vi "Global_ACT Write_Data Out.vi"() -> ()   [LabVIEW 2017, in "Claw.lvlib"]
uses:
  Claw.lvlib
  <vilib>/Rock Robotics/WPI/Solenoid/WPI_SolenoidValue.ctl
  TypeDef/CLUSTER_Two Motor Output.ctl
  CLUSTER_Limit_Switch_Output.ctl
panel:
  in  "Claw_ACT_Limit_Switch":T1
  in  "Claw_ACT_Claw_Motors":T2
  in  "Claw_ACT_Piston_Output":T3
  # "The Names of the Data items in the Global Variable MUST describe who the Single Writer is\nNaming Convention of all Data Items is:   \nLib Name_Loop Name (SM or SEN or ACT)_Data Name\nExamples:\nDrive_ACT_X axis\nGameController_SEN_JoystickLeft\nHopper_SM_AgitatorSpeed"
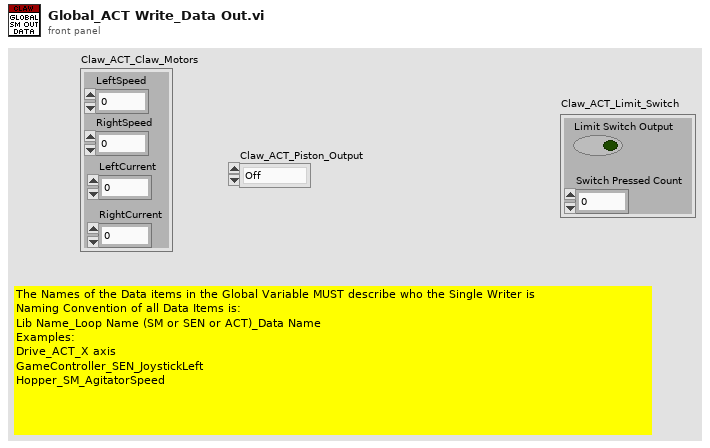
[diagram p1: front panel]
types:
  T1 = typedef "Claw.lvlib/CLUSTER_Limit_Switch_Output.ctl" = cluster{"Limit Switch Output":bool, "Switch Pressed Count":i32}
  T2 = typedef "CLUSTER_Two Motor Output.ctl" = cluster{"LeftSpeed":dbl, "RightSpeed":dbl, "LeftCurrent":dbl, "RightCurrent":dbl}
  T3 = typedef "WPI_SolenoidValue.ctl" = enum16{"Off", "On", "Forward", "Reverse"}
diagram:
